vi "MFP3D Driver.vi"() -> ()   [LabVIEW 2016]
uses:
  Asylum/subVIs/Driver Variables.vi
  subVIs/Global Variables.vi
panel:
  in  "Data Queue":refnum<queue>
  in  "Amplifier Setting":dbl=-15.0
  in  "Interpolation Distance (µm)":dbl=0.1
  in  "Background Image":refnum<vi>
  in  "Inkscape File (.svg)":refnum<vi>
  in  "Run":refnum<vi>
  in  "Abort":refnum<vi>
  in  "Lithography Data":T1(array[cluster])
  in  "Display Wave":bool
  in  "PID Close":bool
  in  "Withdraw Tip When Done":bool=TRUE
  in  "Move Z Set Point":dbl=-1.3
  in  "Z Set Point":dbl=-0.05
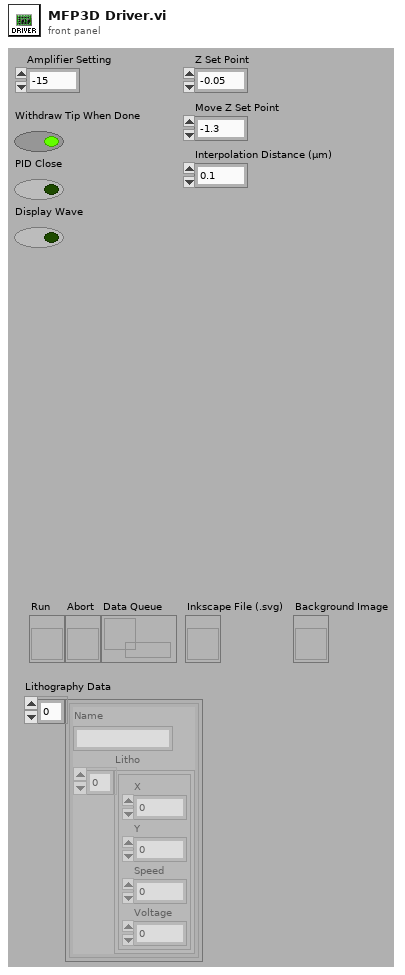
[diagram p1: front panel]
types:
  T1 = cluster{"Name":string, "Litho":cluster{"X":dbl, "Y":dbl, "Speed":dbl, "Voltage":dbl}[]}[]
  T2 = cluster{"X Offset (µm)":dbl, "Y Offset (µm)":dbl}
  T3 = cluster{"Coordinate":cluster{"X":dbl, "Y":dbl}, "Speed":dbl, "Voltage":dbl, "RGB Value":dbl, "Name":string}[][]
  T4 = cluster{"Array":cluster{"Coordinate":cluster{"X":dbl, "Y":dbl}, "Speed":dbl, "Voltage":dbl, "RGB Value":dbl, "Name":string}[][], "Size":cluster{"Width":dbl, "Height":dbl}, cluster{"X Offset (µm)":dbl, "Y Offset (µm)":dbl}, "Interpolation Distance (µm)":dbl, "Z Set Point":dbl, "Move Z Set Point":dbl, "PID Close":bool, "Display Wave":bool, "Run":refnum<vi>}
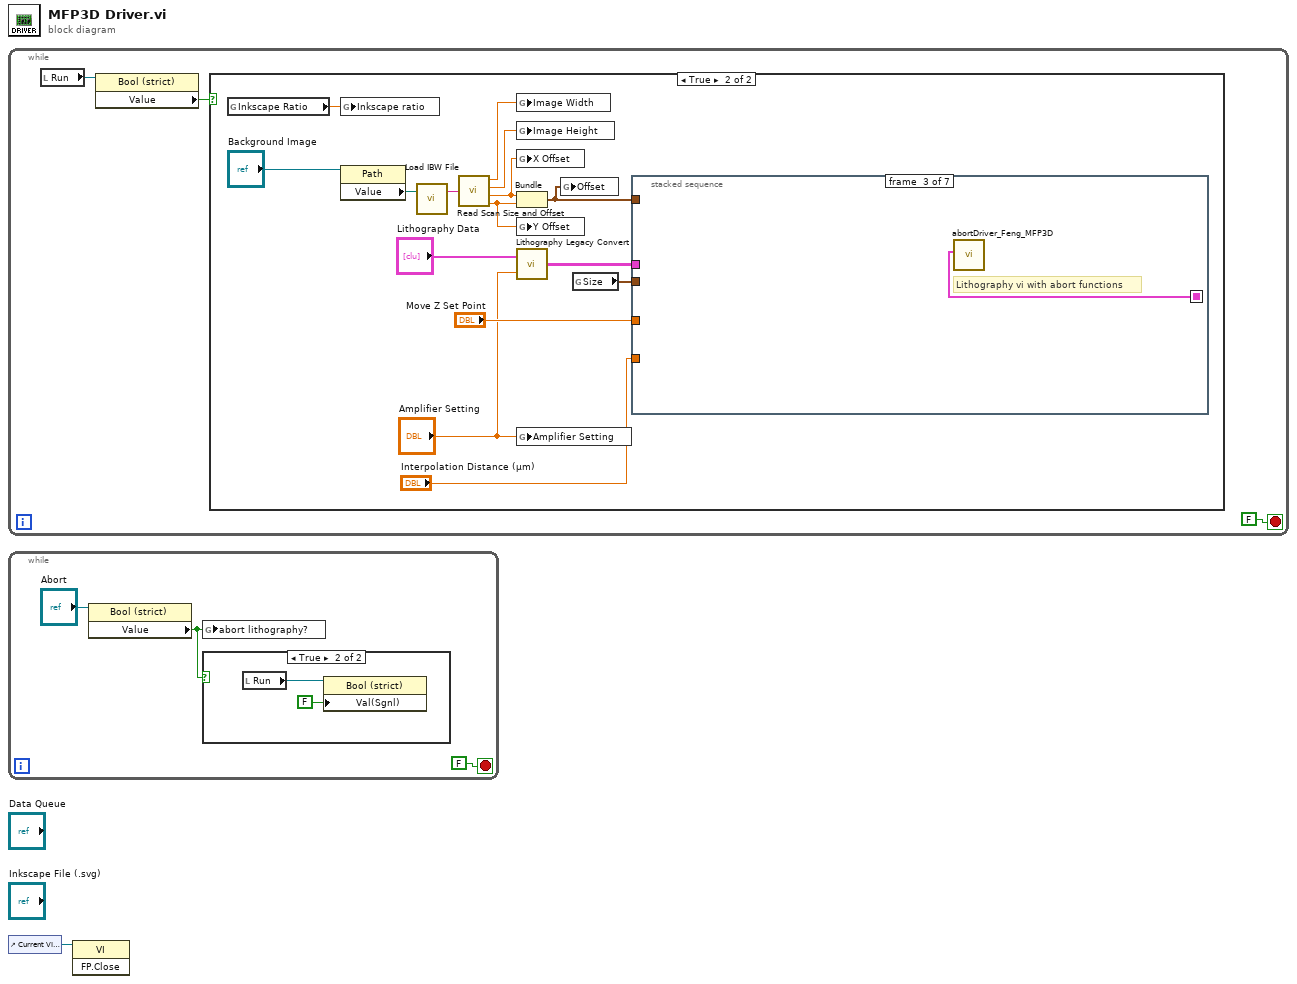
[diagram p0: block diagram]
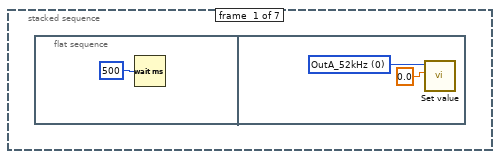
[diagram p3: hidden frame]
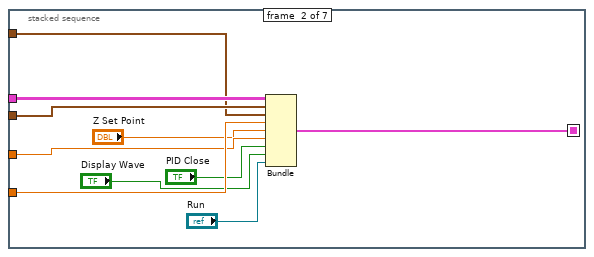
[diagram p4: hidden frame]
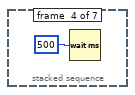
[diagram p5: hidden frame]
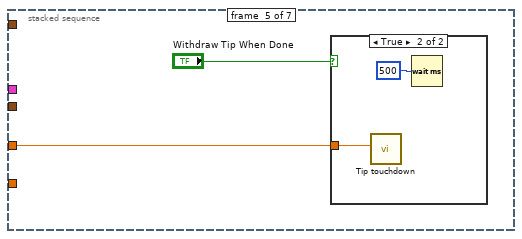
[diagram p6: hidden frame]
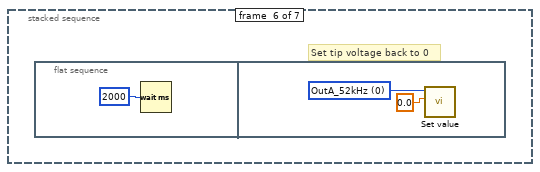
[diagram p8: hidden frame]
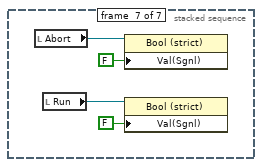
[diagram p9: hidden frame]
diagram:
  n1 = while {
    stop <- FALSE stop-if-true
    n2 = local read "Run"() -> (w3:refnum<vi>)
    n3 = property class="Bool (strict)"(reference=w3) -> ("Value"=w2:bool)  [unwired: 1 in, 2 out]
    n4 = case shown="True" w2 {
      frame False {
      }
      frame True {
        n5 = global read "Global Variables.vi" "Inkscape Ratio"() -> (w10:dbl)
        n6 = global write "Driver Variables.vi" "Inkscape ratio"(w10) -> ()
        n7 = property class="Path"(reference="Background Image") -> ("Value"=w7:path)  [unwired: 1 in, 2 out]
        n8 = call "Load IBW File.vi"("file path (dialog if empty)"=w7) -> ("Wave Note"=w6:string)  [unwired: 1 in, 1 out]
        n9 = call "Read Scan Size and Offset.vi"("Read in the string file"=w6) -> ("X Range (µm)"=w15:dbl, "Y Range (µm)"=w14:dbl, "X Offset (µm)"=w13:dbl, "Y Offset (µm)"=w12:dbl)  [unwired: 4 in]
        n10 = global write "Driver Variables.vi" "Image Width"(w15) -> ()
        n11 = global write "Driver Variables.vi" "Image Height"(w14) -> ()
        n12 = global write "Driver Variables.vi" "X Offset"(w13) -> ()
        n13 = Bundle("X Offset (µm)"=w13, "Y Offset (µm)"=w12) -> (w11:T2)  [unwired: 1 in]
        n14 = global write "Driver Variables.vi" "Y Offset"(w12) -> ()
        n15 = call "Lithography Legacy Convert.vi"("Amplifier Setting"="Amplifier Setting", "Lithography Data"="Lithography Data") -> ("Array"=w9:T3)
        n16 = global write "Driver Variables.vi" "Amplifier Setting"("Amplifier Setting") -> ()
        n17 = global write "Global Variables.vi" "Offset"(w11) -> ()
        n18 = global read "Global Variables.vi" "Size"() -> (w18:cluster{"Width":dbl, "Height":dbl})
        n19 = stacked-sequence {
          seq-local: [_ w27 _ _ _ _ _] -> [_ _ w33 _ _ _ _]
          tunnel: w9 -> [_ w32 _ _ _ _ _]
          tunnel: w18 -> [_ w31 _ _ _ _ _]
          tunnel: "Interpolation Distance (µm)" -> [_ w29 _ _ _ _ _]
          tunnel: w11 -> [_ w30 _ _ _ _ _]
          tunnel: "Move Z Set Point" -> [_ w28 _ _ w36 _ _]
          frame #0 {
            n20 = flat-sequence {
              frame #0 {
                n21 = Wait (ms)(milliseconds to wait=u32 500) -> ()  [unwired: 1 out]
              }
              frame #1 {
                w22 = u16 0 items=["OutA_52kHz", "OutB_52kHz", "OutC_78Hz", "PiezoX", "PiezoY", "PiezoZ", "DDS_Frequency1", "DDS_Frequency2", "DDS_Amplitude1", "DDS_Amplitude2", "DDS_DCOffset", "\"Setpoint%PIDSLoop.3\"", "\"Setpoint%PIDSLoop.4\"", ""] ("Output")
                n22 = call "Set value.vi"("Value"=0.0, "Output"=w22) -> ()  [unwired: 9 in, 1 out]
              }
            }
          }
          frame #1 {
            n23 = Bundle("Array"=w32, "Size"=w31, w30, "Interpolation Distance (µm)"=w29, "Z Set Point"="Z Set Point", "Move Z Set Point"=w28, "PID Close"="PID Close", "Display Wave"="Display Wave", "Run"="Run") -> (w27:T4)  [unwired: 1 in]
          }
          frame #2 {
            # "Lithography vi with abort functions"
            n24 = call "abortDriver_Feng_MFP3D.vi"("litho comm"=w33) -> ()  [unwired: 11 in]
          }
          frame #3 {
            n25 = Wait (ms)(milliseconds to wait=u32 500) -> ()  [unwired: 1 out]
          }
          frame #4 {
            n26 = case shown="True" "Withdraw Tip When Done" {
              tunnel: w36 -> [_ w37]
              frame False {
              }
              frame True {
                n27 = call "Tip touchdown.vi"("Z SetPoint"=w37) -> ()  [unwired: 11 out]
                n28 = Wait (ms)(milliseconds to wait=u32 500) -> ()  [unwired: 1 out]
              }
            }
          }
          frame #5 {
            # "Set tip voltage back to 0"
            n29 = flat-sequence {
              frame #0 {
                n30 = Wait (ms)(milliseconds to wait=u32 2000) -> ()  [unwired: 1 out]
              }
              frame #1 {
                w41 = u16 0 items=["OutA_52kHz", "OutB_52kHz", "OutC_78Hz", "PiezoX", "PiezoY", "PiezoZ", "DDS_Frequency1", "DDS_Frequency2", "DDS_Amplitude1", "DDS_Amplitude2", "DDS_DCOffset", "\"Setpoint%PIDSLoop.3\"", "\"Setpoint%PIDSLoop.4\"", ""] ("Output")
                n31 = call "Set value.vi"("Value"=0.0, "Output"=w41) -> ()  [unwired: 9 in, 1 out]
              }
            }
          }
          frame #6 {
            n32 = local read "Abort"() -> (w42:refnum<vi>)
            n33 = local read "Run"() -> (w45:refnum<vi>)
            n34 = property class="Bool (strict)"(reference=w42, "Val(Sgnl)"=FALSE ("Value (Signaling)")) -> ()  [unwired: 1 in, 2 out]
            n35 = property class="Bool (strict)"(reference=w45, "Val(Sgnl)"=FALSE ("Value (Signaling)")) -> ()  [unwired: 1 in, 2 out]
          }
        }
      }
    }
  }
  n36 = while {
    stop <- FALSE stop-if-true
    n37 = property class="Bool (strict)"(reference="Abort") -> ("Value"=w46:bool)  [unwired: 1 in, 2 out]
    n38 = global write "Driver Variables.vi" "abort lithography?"(w46) -> ()
    n39 = case shown="True" w46 {
      frame False {
      }
      frame True {
        n40 = local read "Run"() -> (w50:refnum<vi>)
        n41 = property class="Bool (strict)"(reference=w50, "Val(Sgnl)"=FALSE ("Value (Signaling)")) -> ()  [unwired: 1 in, 2 out]
      }
    }
  }
  n42 = control-ref of="Current VI Reference"() -> (w1:refnum<vi>)
  n43 = invoke class="VI" method="FP.Close"(reference=w1) -> ()  [unwired: 2 in, 3 out]
